vi "Teleop.vi"(10 "Match Info":T1={"Autonomous Elapsed Seconds"=0.0, "TeleOp Elapsed Seconds"=0.0, "Disabled Elapsed Seconds"=0.0, "Visited Autonomous"=FALSE, "Visited TeleOp"=FALSE, "Visited Disabled"=FALSE, "Autonomous Settings"={"Autonomous Style"=enum."Independent", "VI Refnum"=refnum}}, 11 "Call Context":T2) -> ()   [LabVIEW 2016]
doc: "This VI is called for each TeleOp packet received from the DS where the robot is not disabled. It is often used to read from the joysticks and update I/O or to update setpoints for timed control loops. It should complete and return within 20 milliseconds or it may miss DS packets."
uses:
  <vilib>/Rock Robotics/WPI/DriverStation/WPI_DriverStationDerivedRobotMode.ctl
  <vilib>/Rock Robotics/WPI/DriverStation/WPI_DriverStationMatch Info.ctl
  Robot Global Data.vi
  <vilib>/Rock Robotics/WPI/RobotDrive/WPI_RobotDriveArcadeDrive_Standard(NoSaturation).vi
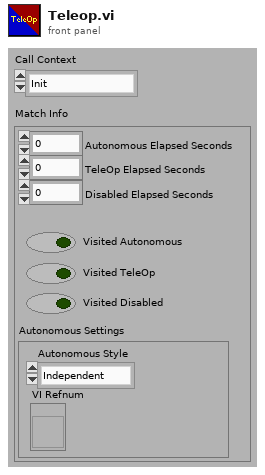
[diagram p1: front panel]
types:
  T1 = typedef "WPI_DriverStationMatch Info.ctl" = cluster{"Autonomous Elapsed Seconds":dbl, "TeleOp Elapsed Seconds":dbl, "Disabled Elapsed Seconds":dbl, "Visited Autonomous":bool, "Visited TeleOp":bool, "Visited Disabled":bool, "Autonomous Settings":cluster{"Autonomous Style":enum16{"Iterative", "Independent"}, "VI Refnum":refnum<vi>}}
  T2 = typedef "WPI_DriverStationDerivedRobotMode.ctl" = enum16{"Init", "Execute", "Stop"}
  T3 = typedef "WPI_RobotDriveDevRef.ctl" = cluster{"DevStatus":errorcluster, "Motors[]":T4[], "Square Inputs":bool, "Max Output":dbl}
  T4 = typedef "WPI_MotorControlDeviceRef.ctl" = cluster{"DeviceStatus":errorcluster, "Type":T5, "PWM":cluster{"PWM Channel":T6, "DeadBand":T7}, "CAN":cluster{"Device Number":u8, "SetOutput VI Ref":variant, "GetOutput VI Ref":variant, "Enable VI Ref":variant, "Disable VI Ref":variant, "Data":variant}, "Invert":bool}
  T5 = typedef "WPI_MotorControlType.ctl" = enum16{"PWM", "CAN"}
  T6 = typedef "FPGA_DIOPWMChannel.ctl" = enum8{"PWM 0", "PWM 1", "PWM 2", "PWM 3", "PWM 4", "PWM 5", "PWM 6", "PWM 7", "PWM 8", "PWM 9", "PWM MXP 0", "PWM MXP 1", "PWM MXP 2", "PWM MXP 3", "PWM MXP 4", "PWM MXP 5", "PWM MXP 6", "PWM MXP 7", "PWM MXP 8", "PWM MXP 9", "Invalid"}
  T7 = typedef "WPI_PWMDeadband.ctl" = cluster{"Name":string, "maxPositivePwm":i32, "minPositivePwm":i32, "centerPwm":i32, "maxNegativePwm":i32, "minNegativePwm":i32, "angularRange":u16}
  T8 = enum16{"Init", "Tank drive", "Right Arcade", "Left Arcade", "Forward", "Vision Alignment", "Stop"}
  T9 = enum16{"Init", "Tank Drive", "Left Arcade", "Right Arcade", "Forward", "Vision Alignment", "Climb", "Stop"}
  T10 = enum16{"Init", "Tank Drive", "Left Arcade", "Right Arcade", "Forward", "Back", "Vision Alignment", "Climb", "Stop"}
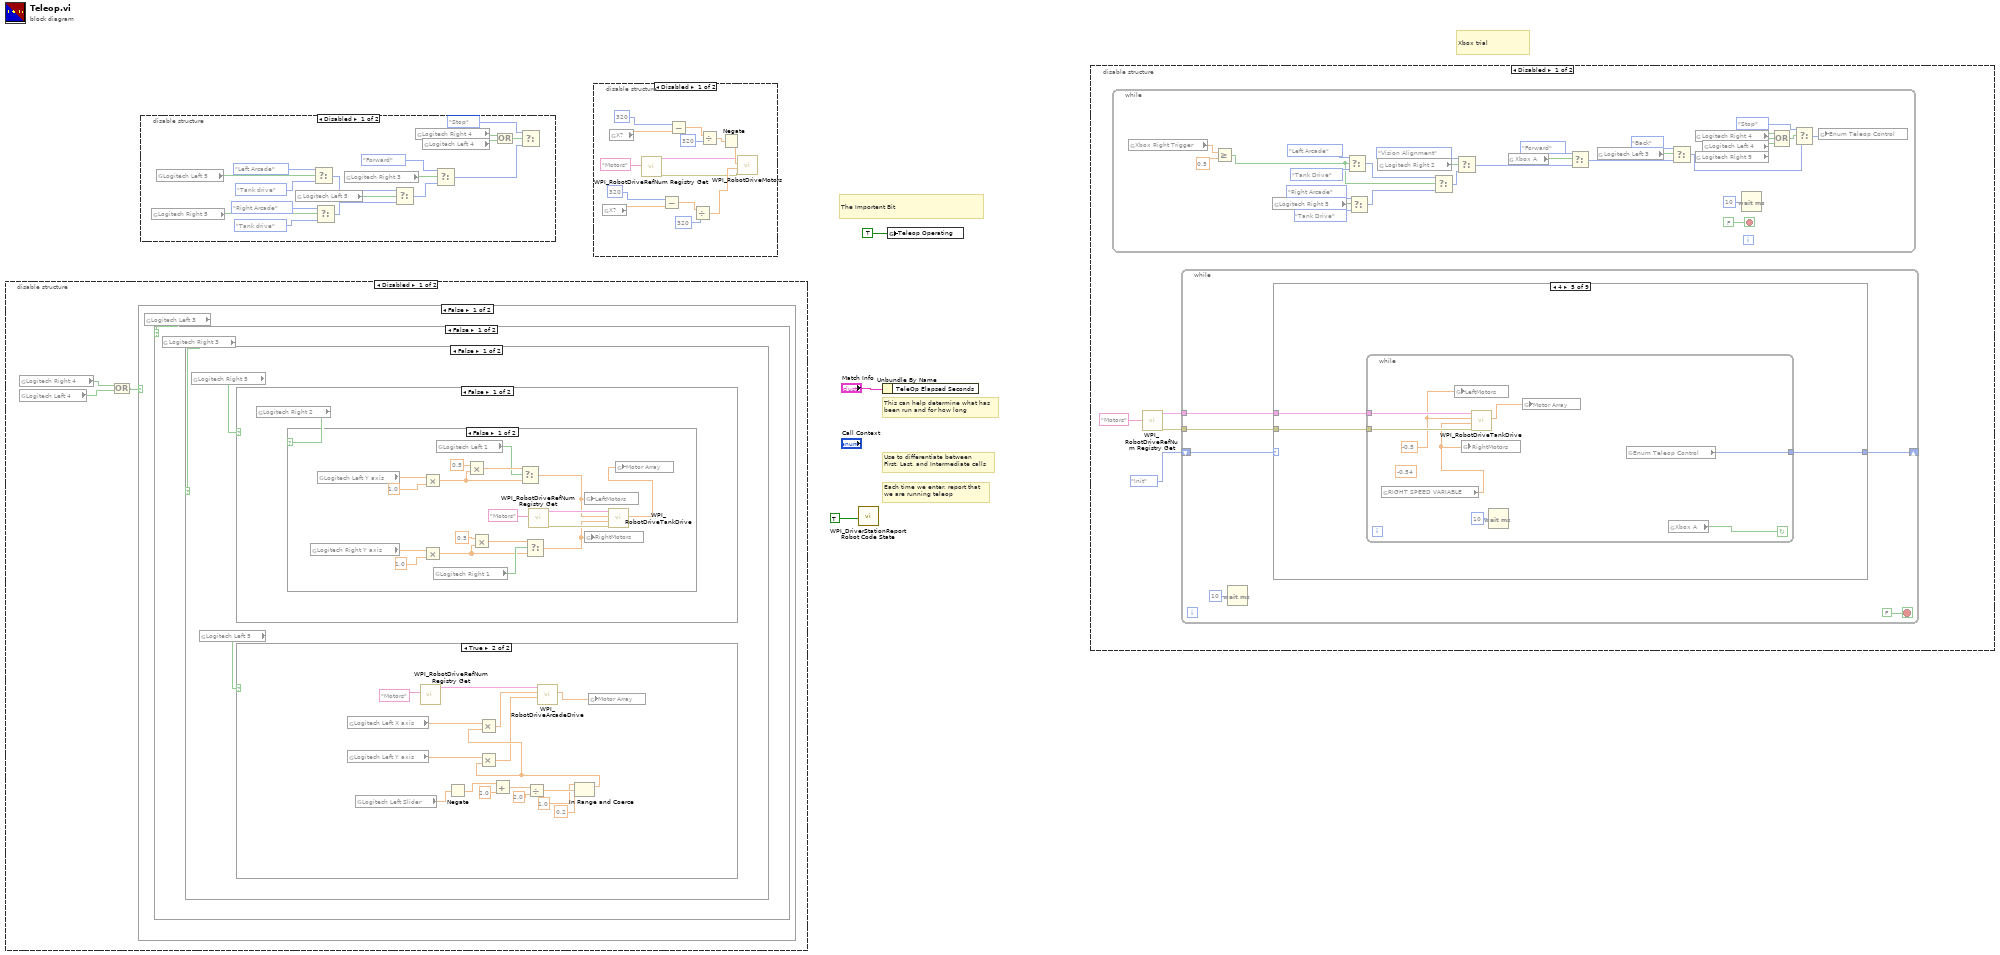
[diagram p0: block diagram]
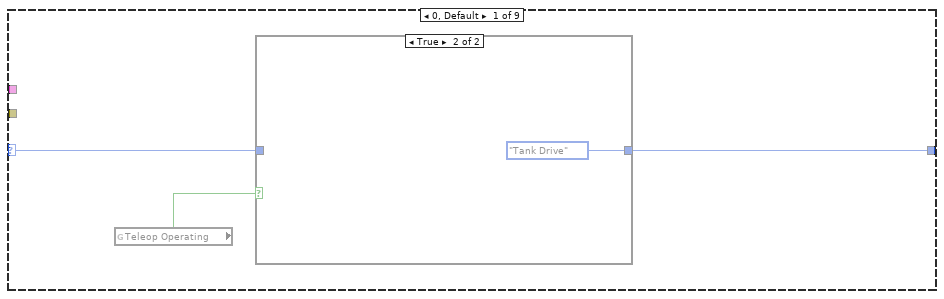
[diagram p2: hidden frame]
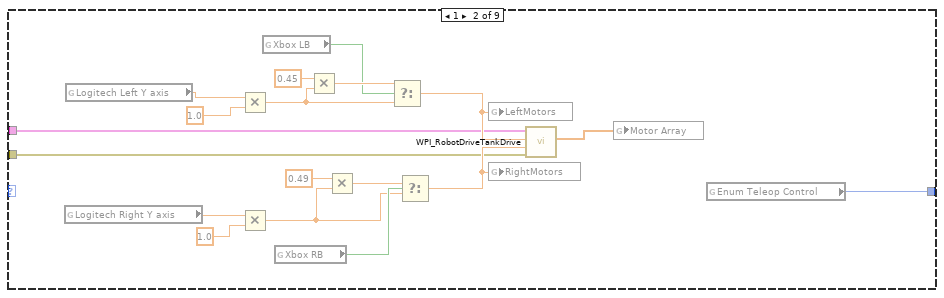
[diagram p4: hidden frame]
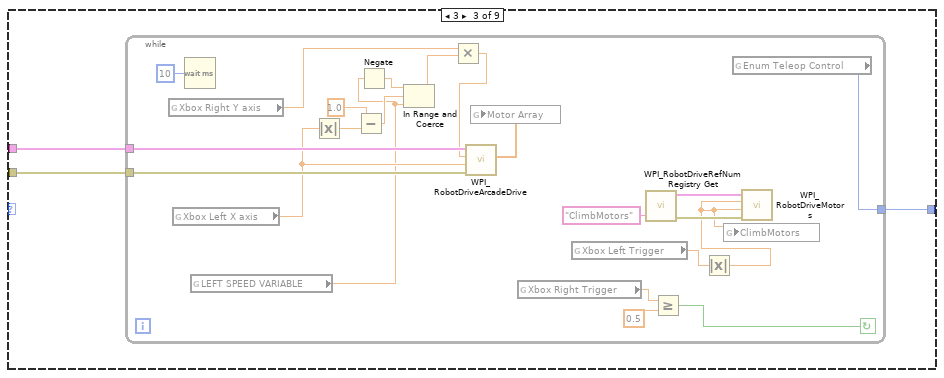
[diagram p5: hidden frame]
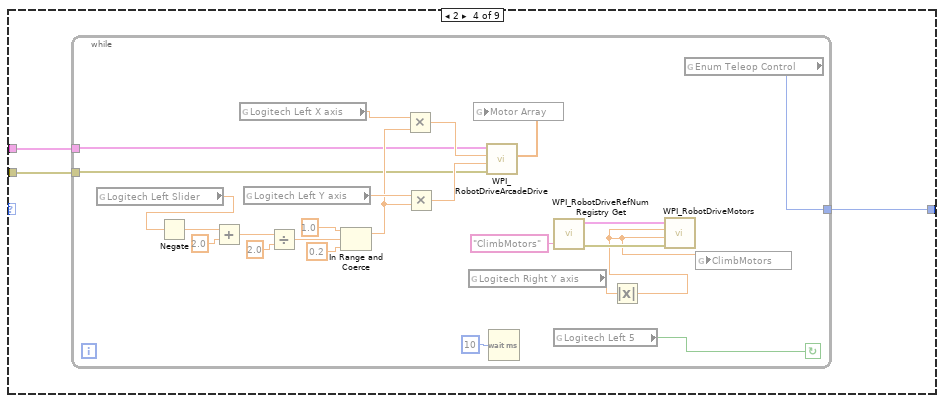
[diagram p6: hidden frame]
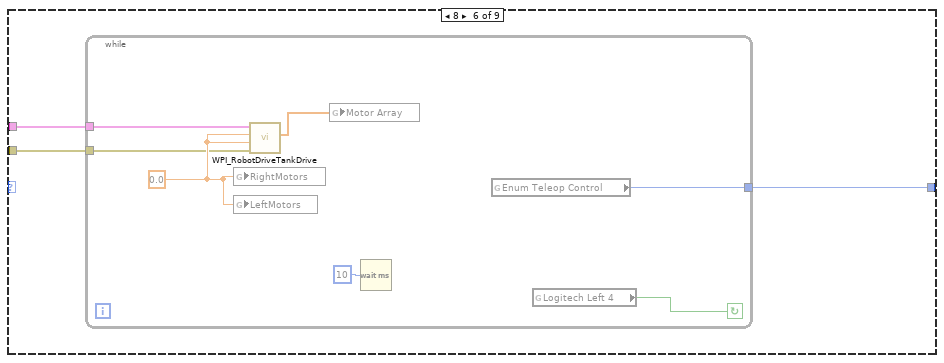
[diagram p7: hidden frame]
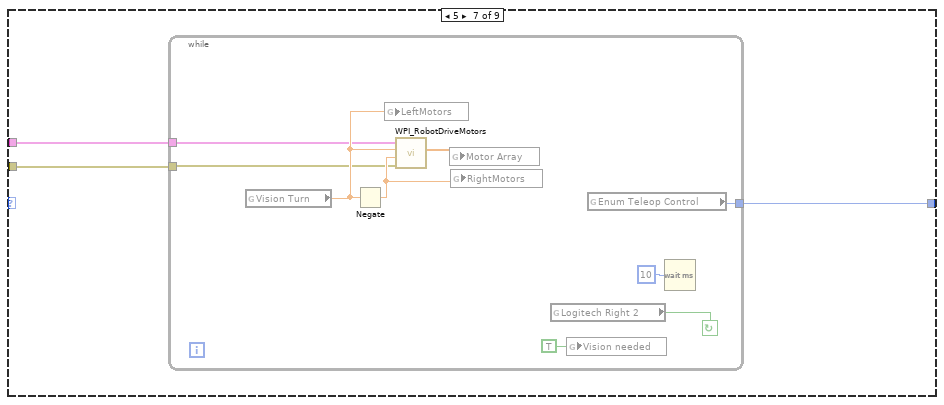
[diagram p8: hidden frame]
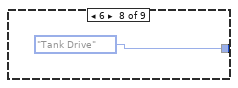
[diagram p9: hidden frame]
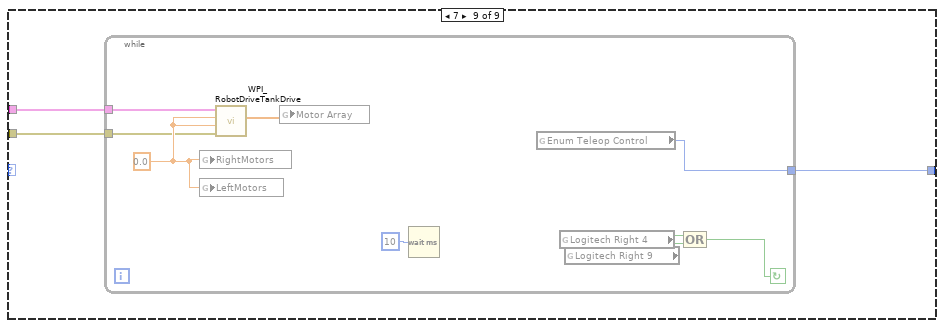
[diagram p10: hidden frame]
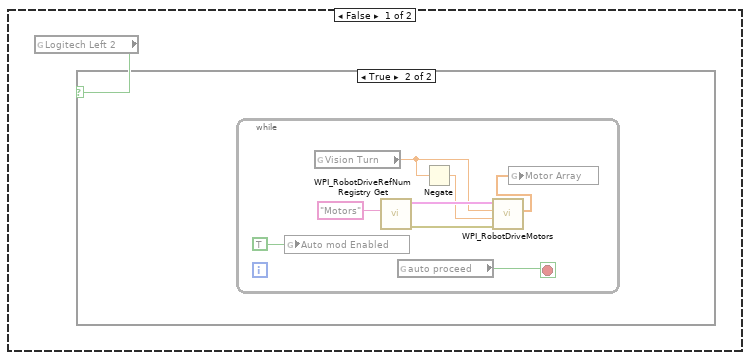
[diagram p12: hidden frame]
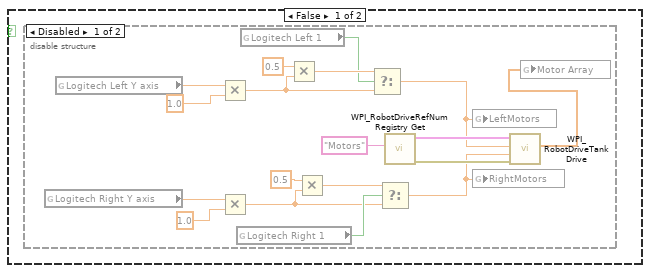
[diagram p13: hidden frame]
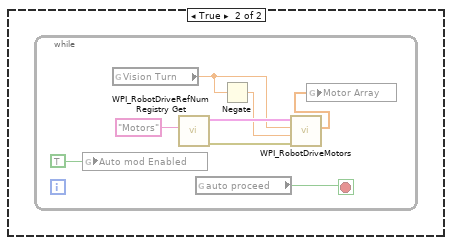
[diagram p15: hidden frame]
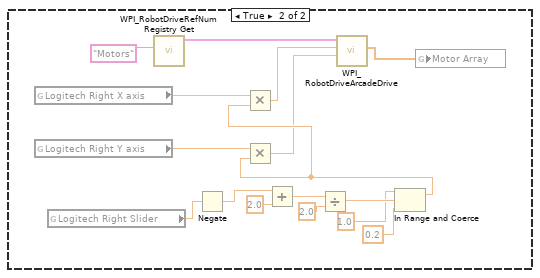
[diagram p16: hidden frame]
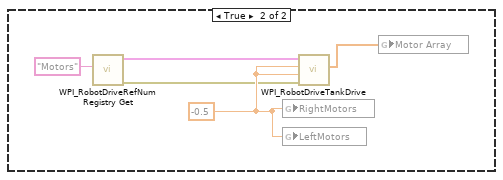
[diagram p17: hidden frame]
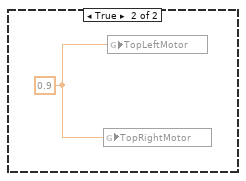
[diagram p18: hidden frame]
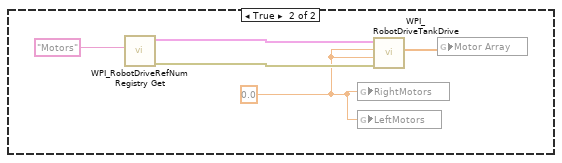
[diagram p19: hidden frame]
diagram:
  # "Xbox trial"
  # "The Importent Bit"
  # "Each time we enter, report that\nwe are running teleop"
  # "Use to differentiate between\nFirst, Last, and Intermediate calls"
  # "This can help determine what has\nbeen run and for how long"
  n1 = disable-structure shown="Disabled" {
    frame Disabled {
      n2 = global read "Robot Global Data.vi" "Logitech Right 4"() -> (w4:bool)
      n3 = global read "Robot Global Data.vi" "Logitech Left 4"() -> (w6:bool)
      n4 = Compound Arithmetic op=OR(w4, w6) -> (w5:bool)
      n5 = case shown="False" w5 {
        frame False {
          n6 = global read "Robot Global Data.vi" "Logitech Left 3"() -> (w7:bool)
          n7 = case shown="False" w7 {
            frame False {
              n8 = global read "Robot Global Data.vi" "Logitech Right 3"() -> (w8:bool)
              n9 = case shown="False" w8 {
                frame False {
                  n10 = global read "Robot Global Data.vi" "Logitech Right 5"() -> (w10:bool)
                  n11 = global read "Robot Global Data.vi" "Logitech Left 5"() -> (w9:bool)
                  n12 = case shown="False" w10 {
                    frame False {
                      n13 = global read "Robot Global Data.vi" "Logitech Right 2"() -> (w54:bool)
                      n14 = case shown="False" w54 {
                        frame False {
                          n15 = global read "Robot Global Data.vi" "Logitech Right Y axis"() -> (w66:dbl)
                          n16 = global read "Robot Global Data.vi" "Logitech Left Y axis"() -> (w69:dbl)
                          n17 = Multiply(x=w69, y=1.0) -> (x*y=w63:dbl)
                          n18 = Multiply(x=w66, y=1.0) -> (x*y=w59:dbl)
                          n19 = global read "Robot Global Data.vi" "Logitech Right 1"() -> (w60:bool)
                          n20 = global read "Robot Global Data.vi" "Logitech Left 1"() -> (w58:bool)
                          n21 = Multiply(x=0.5 ("y"), y=w63) -> (x*y=w64:dbl)
                          n22 = Multiply(x=0.5 ("y"), y=w59) -> (x*y=w62:dbl)
                          n23 = Select(t=w64, s=w58, f=w63) -> (s? t:f=w57:dbl)
                          n24 = Select(t=w62, s=w60, f=w59) -> (s? t:f=w56:dbl)
                          n25 = call <vilib>:"WPI_RobotDriveRefNum Registry Get.vi"("refnum name"="Motors") -> ("error out"=w71:errorcluster, "RobotDriveDevRef"=w72:T3)  [unwired: 9 in]
                          n26 = global write "Robot Global Data.vi" "LeftMotors"(w57) -> ()
                          n27 = global write "Robot Global Data.vi" "RightMotors"(w56) -> ()
                          n28 = call <vilib>:"WPI_RobotDriveTankDrive.vi"("error in (no error)"=w71, "Right axis value"=w56, "Left axis value"=w57, "RobotDriveDevRef"=w72) -> ("Motor Values"=w55:dbl[])  [unwired: 5 in, 2 out]
                          n29 = global write "Robot Global Data.vi" "Motor Array"(w55) -> ()
                        }
                        frame True {
                          n30 = while {
                            stop <- w74 stop-if-true
                            n31 = global write "Robot Global Data.vi" "Auto mod Enabled"(TRUE ("Auto mod Enabled")) -> ()
                            n32 = global read "Robot Global Data.vi" "Vision Turn"() -> (w77:dbl)
                            n33 = call <vilib>:"WPI_RobotDriveRefNum Registry Get.vi"("refnum name"="Motors") -> ("error out"=w78:errorcluster, "RobotDriveDevRef"=w79:T3)  [unwired: 9 in]
                            n34 = global read "Robot Global Data.vi" "auto proceed"() -> (w74:bool)
                            n35 = Negate(x=w77) -> (-x=w76:dbl)
                            n36 = call <vilib>:"WPI_RobotDriveMotors.vi"("error in (no error)"=w78, "RightSpeed"=w76, "LeftSpeed"=w77, "RobotDriveDevRef"=w79) -> ("Motor Values"=w73:dbl[])  [unwired: 7 out]
                            n37 = global write "Robot Global Data.vi" "Motor Array"(w73) -> ()
                          }
                        }
                      }
                    }
                    frame True {
                      n38 = global read "Robot Global Data.vi" "Logitech Right X axis"() -> (w88:dbl)
                      n39 = global read "Robot Global Data.vi" "Logitech Right Y axis"() -> (w87:dbl)
                      n40 = global read "Robot Global Data.vi" "Logitech Right Slider"() -> (w92:dbl)
                      n41 = call <vilib>:"WPI_RobotDriveRefNum Registry Get.vi"("refnum name"="Motors") -> ("RobotDriveDevRef"=w83:T3)  [unwired: 9 in, 1 out]
                      n42 = Negate(x=w92) -> (-x=w91:dbl)
                      n43 = Add(x=w91, y=2.0) -> (x+y=w85:dbl)
                      n44 = Divide(x=w85, y=2.0) -> (x/y=w95:dbl)
                      n45 = In Range and Coerce(upper limit=1.0, x=w95, lower limit=0.2) -> (coerced(x)=w96:dbl)  [unwired: 1 out]
                      n46 = Multiply(x=w88, y=w96) -> (x*y=w89:dbl)
                      n47 = Multiply(x=w87, y=w96) -> (x*y=w90:dbl)
                      n48 = call-poly <vilib>:"WPI_RobotDriveArcadeDrive.vi"("Y axis value"=w90, "X axis value"=w89, "RobotDriveDevRef"=w83) -> ("Motor Values"=w81:dbl[])  [unwired: 6 in, 2 out]
                      n49 = global write "Robot Global Data.vi" "Motor Array"(w81) -> ()
                    }
                  }
                  n50 = case shown="True" w9 {
                    frame False {
                      n51 = global read "Robot Global Data.vi" "Logitech Left 2"() -> (w11:bool)
                      n52 = case shown="True" w11 {
                        frame False {
                          n53 = disable-structure shown="Disabled" {
                            frame Disabled {
                              n54 = global read "Robot Global Data.vi" "Logitech Right Y axis"() -> (w23:dbl)
                              n55 = global read "Robot Global Data.vi" "Logitech Left Y axis"() -> (w26:dbl)
                              n56 = Multiply(x=w26, y=1.0) -> (x*y=w20:dbl)
                              n57 = Multiply(x=w23, y=1.0) -> (x*y=w16:dbl)
                              n58 = global read "Robot Global Data.vi" "Logitech Right 1"() -> (w17:bool)
                              n59 = global read "Robot Global Data.vi" "Logitech Left 1"() -> (w15:bool)
                              n60 = Multiply(x=0.5 ("y"), y=w20) -> (x*y=w21:dbl)
                              n61 = Multiply(x=0.5 ("y"), y=w16) -> (x*y=w19:dbl)
                              n62 = Select(t=w21, s=w15, f=w20) -> (s? t:f=w14:dbl)
                              n63 = Select(t=w19, s=w17, f=w16) -> (s? t:f=w13:dbl)
                              n64 = call <vilib>:"WPI_RobotDriveRefNum Registry Get.vi"("refnum name"="Motors") -> ("error out"=w28:errorcluster, "RobotDriveDevRef"=w29:T3)  [unwired: 9 in]
                              n65 = global write "Robot Global Data.vi" "LeftMotors"(w14) -> ()
                              n66 = global write "Robot Global Data.vi" "RightMotors"(w13) -> ()
                              n67 = call <vilib>:"WPI_RobotDriveTankDrive.vi"("error in (no error)"=w28, "Right axis value"=w13, "Left axis value"=w14, "RobotDriveDevRef"=w29) -> ("Motor Values"=w12:dbl[])  [unwired: 5 in, 2 out]
                              n68 = global write "Robot Global Data.vi" "Motor Array"(w12) -> ()
                            }
                            frame Enabled {
                            }
                          }
                        }
                        frame True {
                          n69 = while {
                            stop <- w31 stop-if-true
                            n70 = global write "Robot Global Data.vi" "Auto mod Enabled"(TRUE ("Auto mod Enabled")) -> ()
                            n71 = global read "Robot Global Data.vi" "Vision Turn"() -> (w34:dbl)
                            n72 = call <vilib>:"WPI_RobotDriveRefNum Registry Get.vi"("refnum name"="Motors") -> ("error out"=w35:errorcluster, "RobotDriveDevRef"=w36:T3)  [unwired: 9 in]
                            n73 = global read "Robot Global Data.vi" "auto proceed"() -> (w31:bool)
                            n74 = Negate(x=w34) -> (-x=w33:dbl)
                            n75 = call <vilib>:"WPI_RobotDriveMotors.vi"("error in (no error)"=w35, "RightSpeed"=w33, "LeftSpeed"=w34, "RobotDriveDevRef"=w36) -> ("Motor Values"=w30:dbl[])  [unwired: 7 out]
                            n76 = global write "Robot Global Data.vi" "Motor Array"(w30) -> ()
                          }
                        }
                      }
                    }
                    frame True {
                      n77 = global read "Robot Global Data.vi" "Logitech Left X axis"() -> (w45:dbl)
                      n78 = global read "Robot Global Data.vi" "Logitech Left Y axis"() -> (w44:dbl)
                      n79 = global read "Robot Global Data.vi" "Logitech Left Slider"() -> (w49:dbl)
                      n80 = call <vilib>:"WPI_RobotDriveRefNum Registry Get.vi"("refnum name"="Motors") -> ("RobotDriveDevRef"=w40:T3)  [unwired: 9 in, 1 out]
                      n81 = Negate(x=w49) -> (-x=w48:dbl)
                      n82 = Add(x=w48, y=2.0) -> (x+y=w42:dbl)
                      n83 = Divide(x=w42, y=2.0) -> (x/y=w52:dbl)
                      n84 = In Range and Coerce(upper limit=1.0, x=w52, lower limit=0.2) -> (coerced(x)=w53:dbl)  [unwired: 1 out]
                      n85 = Multiply(x=w45, y=w53) -> (x*y=w46:dbl)
                      n86 = Multiply(x=w44, y=w53) -> (x*y=w47:dbl)
                      n87 = call-poly <vilib>:"WPI_RobotDriveArcadeDrive.vi"("Y axis value"=w47, "X axis value"=w46, "RobotDriveDevRef"=w40) -> ("Motor Values"=w38:dbl[])  [unwired: 6 in, 2 out]
                      n88 = global write "Robot Global Data.vi" "Motor Array"(w38) -> ()
                    }
                  }
                }
                frame True {
                  w101 = -0.5 ("Right axis value")
                  n89 = call <vilib>:"WPI_RobotDriveRefNum Registry Get.vi"("refnum name"="Motors") -> ("error out"=w99:errorcluster, "RobotDriveDevRef"=w100:T3)  [unwired: 9 in]
                  n90 = global write "Robot Global Data.vi" "RightMotors"(w101) -> ()
                  n91 = global write "Robot Global Data.vi" "LeftMotors"(w101) -> ()
                  n92 = call <vilib>:"WPI_RobotDriveTankDrive.vi"("error in (no error)"=w99, "Right axis value"=w101, "Left axis value"=w101, "RobotDriveDevRef"=w100) -> ("Motor Values"=w97:dbl[])  [unwired: 5 in, 2 out]
                  n93 = global write "Robot Global Data.vi" "Motor Array"(w97) -> ()
                }
              }
            }
            frame True {
              w102 = 0.9
              n94 = global write "Robot Global Data.vi" "TopRightMotor"(w102) -> ()
              n95 = global write "Robot Global Data.vi" "TopLeftMotor"(w102) -> ()
            }
          }
        }
        frame True {
          w104 = 0.0 ("Right axis value")
          n96 = call <vilib>:"WPI_RobotDriveRefNum Registry Get.vi"("refnum name"="Motors") -> ("error out"=w106:errorcluster, "RobotDriveDevRef"=w105:T3)  [unwired: 9 in]
          n97 = global write "Robot Global Data.vi" "RightMotors"(w104) -> ()
          n98 = global write "Robot Global Data.vi" "LeftMotors"(w104) -> ()
          n99 = call <vilib>:"WPI_RobotDriveTankDrive.vi"("error in (no error)"=w106, "Right axis value"=w104, "Left axis value"=w104, "RobotDriveDevRef"=w105) -> ("Motor Values"=w103:dbl[])  [unwired: 5 in, 2 out]
          n100 = global write "Robot Global Data.vi" "Motor Array"(w103) -> ()
        }
      }
    }
    frame Enabled {
    }
  }
  n101 = disable-structure shown="Disabled" {
    frame Disabled {
      n102 = global read "Robot Global Data.vi" "Logitech Right 5"() -> (w117:bool)
      n103 = global read "Robot Global Data.vi" "Logitech Left 5"() -> (w118:bool)
      n104 = global read "Robot Global Data.vi" "Logitech Left 5"() -> (w121:bool)
      n105 = Select(t=T8."Left Arcade", s=w118, f=T8."Tank drive") -> (s? t:f=w120:T8)
      n106 = Select(t=T8."Right Arcade", s=w117, f=T8."Tank drive") -> (s? t:f=w119:T8)
      n107 = global read "Robot Global Data.vi" "Logitech Right 3"() -> (w122:bool)
      n108 = Select(t=w120, s=w121, f=w119) -> (s? t:f=w124:T8)
      n109 = global read "Robot Global Data.vi" "Logitech Right 4"() -> (w110:bool)
      n110 = global read "Robot Global Data.vi" "Logitech Left 4"() -> (w112:bool)
      n111 = Select(t=T8."Forward", s=w122, f=w124) -> (s? t:f=w108:T8)
      n112 = Compound Arithmetic op=OR(w110, w112) -> (w111:bool)
      n113 = Select(t=T8."Stop", s=w111, f=w108) -> ()  [unwired: 1 out]
    }
    frame Enabled {
    }
  }
  n114 = disable-structure shown="Disabled" {
    frame Disabled {
      n115 = global read "Robot Global Data.vi" "X?"() -> (w133:dbl)
      n116 = global read "Robot Global Data.vi" "X?"() -> (w125:dbl)
      n117 = call <vilib>:"WPI_RobotDriveRefNum Registry Get.vi"("refnum name"="Motors") -> ("error out"=w129:errorcluster, "RobotDriveDevRef"=w130:T3)  [unwired: 9 in]
      n118 = Subtract(x=320, y=w133) -> (x-y=w132:dbl)
      n119 = Subtract(x=320, y=w125) -> (x-y=w126:dbl)
      n120 = Divide(x=w132, y=320) -> (x/y=w134:dbl)
      n121 = Divide(x=w126, y=320) -> (x/y=w135:dbl)
      n122 = Negate(x=w135) -> (-x=w136:dbl)
      n123 = call <vilib>:"WPI_RobotDriveMotors.vi"("error in (no error)"=w129, "RightSpeed"=w134, "LeftSpeed"=w136, "RobotDriveDevRef"=w130) -> ()  [unwired: 8 out]
    }
    frame Enabled {
    }
  }
  n124 = call <vilib>:"WPI_DriverStationReport Robot Code State.vi"("TeleOp"=TRUE ("Autonomous")) -> ()  [unwired: 10 in, 1 out]
  n125 = Unbundle By Name("Match Info") -> ()  [unwired: 1 out]
  n126 = global write "Robot Global Data.vi" "Teleop Operating"(TRUE ("Teleop Enabled")) -> ()
  n127 = disable-structure shown="Disabled" {
    frame Disabled {
      n128 = while {
        stop <- FALSE stop-if-true
        n129 = global read "Robot Global Data.vi" "Xbox Right Trigger"() -> (w144:dbl)
        n130 = Greater Or Equal?(x=w144, y=0.5) -> (x >= y?=w143:bool)
        n131 = global read "Robot Global Data.vi" "Logitech Right 5"() -> (w162:bool)
        n132 = Select(t=T9."Left Arcade", s=w143, f=T9."Tank Drive") -> (s? t:f=w153:T9)
        n133 = Select(t=T9."Right Arcade", s=w162, f=T9."Tank Drive") -> (s? t:f=w152:T9)
        n134 = global read "Robot Global Data.vi" "Logitech Right 2"() -> (w163:bool)
        n135 = Select(t=w153, s=w143, f=w152) -> (s? t:f=w160:T9)
        n136 = Select(t=T9."Vision Alignment", s=w163, f=w160) -> (s? t:f=w161:T9)
        n137 = global read "Robot Global Data.vi" "Xbox A"() -> (w164:bool)
        n138 = Select(t=T9."Forward", s=w164, f=w161) -> (s? t:f=w148:T9)
        n139 = global read "Robot Global Data.vi" "Logitech Left 3"() -> (w149:bool)
        n140 = Select(t=T10."Back", s=w149, f=w148) -> (s? t:f=w147:u16)
        n141 = global read "Robot Global Data.vi" "Logitech Right 4"() -> (w165:bool)
        n142 = global read "Robot Global Data.vi" "Logitech Right 9"() -> (w146:bool)
        n143 = global read "Robot Global Data.vi" "Logitech Left 4"() -> (w166:bool)
        n144 = Wait (ms)(milliseconds to wait=u32 10) -> ()  [unwired: 1 out]
        n145 = Compound Arithmetic op=OR(w165, w166, w146) -> (w167:bool)
        n146 = Select(t=T9."Stop", s=w167, f=w147) -> (s? t:f=w168:u16)
        n147 = global write "Robot Global Data.vi" "Enum Teleop Control"(w168) -> ()
      }
      n148 = call <vilib>:"WPI_RobotDriveRefNum Registry Get.vi"("refnum name"="Motors") -> ("error out"=w141:errorcluster, "RobotDriveDevRef"=w142:T3)  [unwired: 9 in]
      n149 = while {
        tunnel: w142 -> [w176]
        tunnel: w141 -> [w175]
        shift-right: [w171] -> _
        shift-left: T9."Init" -> [w172]
        stop <- FALSE stop-if-true
        n150 = Wait (ms)(milliseconds to wait=u32 10) -> ()  [unwired: 1 out]
        n151 = case shown="4" w172 {
          selector: w172 -> [w177 _ _ _ _ _ _ _ _]
          tunnel: w176 -> [_ w184 w202 w227 w253 w265 w275 _ w288]
          tunnel: w175 -> [_ w183 w201 w226 w254 w264 w274 _ w287]
          tunnel: [w178 w182 w200 w225 w252 w263 w273 T9."Tank Drive" w286] -> w171
          frame 0, Default {
            n152 = global read "Robot Global Data.vi" "Teleop Operating"() -> (w179:bool)
            n153 = case shown="True" w179 {
              tunnel: [w180 T9."Tank Drive"] -> w178
              tunnel: w177 -> [w180 _]
              frame False {
              }
              frame True {
              }
            }
          }
          frame 1 {
            n154 = global read "Robot Global Data.vi" "Logitech Right Y axis"() -> (w196:dbl)
            n155 = global read "Robot Global Data.vi" "Logitech Left Y axis"() -> (w199:dbl)
            n156 = Multiply(x=w199, y=1.0) -> (x*y=w193:dbl)
            n157 = Multiply(x=w196, y=1.0) -> (x*y=w189:dbl)
            n158 = global read "Robot Global Data.vi" "Xbox LB"() -> (w188:bool)
            n159 = global read "Robot Global Data.vi" "Xbox RB"() -> (w190:bool)
            n160 = Multiply(x=0.45 ("y"), y=w193) -> (x*y=w194:dbl)
            n161 = Multiply(x=0.49 ("y"), y=w189) -> (x*y=w192:dbl)
            n162 = Select(t=w194, s=w188, f=w193) -> (s? t:f=w187:dbl)
            n163 = Select(t=w192, s=w190, f=w189) -> (s? t:f=w186:dbl)
            n164 = global write "Robot Global Data.vi" "LeftMotors"(w187) -> ()
            n165 = global write "Robot Global Data.vi" "RightMotors"(w186) -> ()
            n166 = call <vilib>:"WPI_RobotDriveTankDrive.vi"("error in (no error)"=w183, "Right axis value"=w186, "Left axis value"=w187, "RobotDriveDevRef"=w184) -> ("Motor Values"=w185:dbl[])  [unwired: 5 in, 2 out]
            n167 = global write "Robot Global Data.vi" "Motor Array"(w185) -> ()
            n168 = global read "Robot Global Data.vi" "Enum Teleop Control"() -> (w182:u16)
          }
          frame 3 {
            n169 = while {
              tunnel: w202 -> [w223]
              tunnel: w201 -> [w222]
              tunnel: [w220] -> w200
              stop <- w203 continue-if-true
              n170 = global read "Robot Global Data.vi" "Xbox Right Y axis"() -> (w215:dbl)
              n171 = global read "Robot Global Data.vi" "Xbox Left X axis"() -> (w219:dbl)
              n172 = Wait (ms)(milliseconds to wait=u32 10) -> ()  [unwired: 1 out]
              n173 = global read "Robot Global Data.vi" "LEFT SPEED VARIABLE"() -> (w211:dbl)
              n174 = Absolute Value(x=w219) -> (abs(x)=w218:dbl)
              n175 = Subtract(x=1.0, y=w218) -> (x-y=w216:dbl)
              n176 = Negate(x=w211) -> (-x=w212:dbl)
              n177 = In Range and Coerce(upper limit=w212, x=w216, lower limit=w211) -> (coerced(x)=w214:dbl)  [unwired: 1 out]
              n178 = Multiply(x=w215, y=w214) -> (x*y=w213:dbl)
              n179 = call-poly <vilib>:"WPI_RobotDriveArcadeDrive.vi"("error in (no error)"=w222, "Y axis value"=w219, "X axis value"=w213, "RobotDriveDevRef"=w223) -> ("Motor Values"=w224:dbl[])  [unwired: 5 in, 2 out]
              n180 = global write "Robot Global Data.vi" "Motor Array"(w224) -> ()
              n181 = global read "Robot Global Data.vi" "Xbox Right Trigger"() -> (w205:dbl)
              n182 = global read "Robot Global Data.vi" "Xbox Left Trigger"() -> (w207:dbl)
              n183 = call <vilib>:"WPI_RobotDriveRefNum Registry Get.vi"("refnum name"="ClimbMotors") -> ("error out"=w208:errorcluster, "RobotDriveDevRef"=w209:T3)  [unwired: 9 in]
              n184 = Greater Or Equal?(x=w205, y=0.5) -> (x >= y?=w203:bool)
              n185 = Absolute Value(x=w207) -> (abs(x)=w206:dbl)
              n186 = global write "Robot Global Data.vi" "ClimbMotors"(w206) -> ()
              n187 = global read "Robot Global Data.vi" "Enum Teleop Control"() -> (w220:u16)
              n188 = call <vilib>:"WPI_RobotDriveMotors.vi"("error in (no error)"=w208, "RightSpeed"=w206, "LeftSpeed"=w206, "RobotDriveDevRef"=w209) -> ()  [unwired: 8 out]
            }
          }
          frame 2 {
            n189 = while {
              tunnel: w227 -> [w238]
              tunnel: w226 -> [w237]
              tunnel: [w233] -> w225
              stop <- w236 continue-if-true
              n190 = global read "Robot Global Data.vi" "Logitech Left Slider"() -> (w234:dbl)
              n191 = Negate(x=w234) -> (-x=w243:dbl)
              n192 = Add(x=w243, y=2.0) -> (x+y=w249:dbl)
              n193 = global read "Robot Global Data.vi" "Logitech Left X axis"() -> (w246:dbl)
              n194 = global read "Robot Global Data.vi" "Logitech Left Y axis"() -> (w247:dbl)
              n195 = Divide(x=w249, y=2.0) -> (x/y=w240:dbl)
              n196 = In Range and Coerce(upper limit=1.0, x=w240, lower limit=0.2) -> (coerced(x)=w239:dbl)  [unwired: 1 out]
              n197 = Multiply(x=w246, y=w239) -> (x*y=w245:dbl)
              n198 = Multiply(x=w247, y=w239) -> (x*y=w244:dbl)
              n199 = global read "Robot Global Data.vi" "Logitech Right Y axis"() -> (w229:dbl)
              n200 = call-poly <vilib>:"WPI_RobotDriveArcadeDrive.vi"("error in (no error)"=w237, "Y axis value"=w244, "X axis value"=w245, "RobotDriveDevRef"=w238) -> ("Motor Values"=w251:dbl[])  [unwired: 5 in, 2 out]
              n201 = global write "Robot Global Data.vi" "Motor Array"(w251) -> ()
              n202 = Wait (ms)(milliseconds to wait=u32 10) -> ()  [unwired: 1 out]
              n203 = call <vilib>:"WPI_RobotDriveRefNum Registry Get.vi"("refnum name"="ClimbMotors") -> ("error out"=w230:errorcluster, "RobotDriveDevRef"=w231:T3)  [unwired: 9 in]
              n204 = global read "Robot Global Data.vi" "Logitech Left 5"() -> (w236:bool)
              n205 = Absolute Value(x=w229) -> (abs(x)=w228:dbl)
              n206 = call <vilib>:"WPI_RobotDriveMotors.vi"("error in (no error)"=w230, "RightSpeed"=w228, "LeftSpeed"=w228, "RobotDriveDevRef"=w231) -> ()  [unwired: 8 out]
              n207 = global read "Robot Global Data.vi" "Enum Teleop Control"() -> (w233:u16)
              n208 = global write "Robot Global Data.vi" "ClimbMotors"(w228) -> ()
            }
          }
          frame 4 {
            n209 = while {
              tunnel: w254 -> [w261]
              tunnel: w253 -> [w260]
              tunnel: [w258] -> w252
              stop <- w259 continue-if-true
              (unwired) -0.54 ("Right axis value")
              w256 = -0.5 ("Right axis value")
              n210 = global read "Robot Global Data.vi" "RIGHT SPEED VARIABLE"() -> (w255:dbl)
              n211 = global write "Robot Global Data.vi" "LeftMotors"(w256) -> ()
              n212 = global write "Robot Global Data.vi" "RightMotors"(w255) -> ()
              n213 = call <vilib>:"WPI_RobotDriveTankDrive.vi"("error in (no error)"=w261, "Right axis value"=w255, "Left axis value"=w256, "RobotDriveDevRef"=w260) -> ("Motor Values"=w262:dbl[])  [unwired: 5 in, 2 out]
              n214 = Wait (ms)(milliseconds to wait=u32 10) -> ()  [unwired: 1 out]
              n215 = global write "Robot Global Data.vi" "Motor Array"(w262) -> ()
              n216 = global read "Robot Global Data.vi" "Enum Teleop Control"() -> (w258:u16)
              n217 = global read "Robot Global Data.vi" "Xbox A"() -> (w259:bool)
            }
          }
          frame 8 {
            n218 = while {
              tunnel: w264 -> [w270]
              tunnel: w265 -> [w269]
              tunnel: [w268] -> w263
              stop <- w266 continue-if-true
              w271 = 0.0 ("Right axis value")
              n219 = global write "Robot Global Data.vi" "RightMotors"(w271) -> ()
              n220 = global write "Robot Global Data.vi" "LeftMotors"(w271) -> ()
              n221 = call <vilib>:"WPI_RobotDriveTankDrive.vi"("error in (no error)"=w270, "Right axis value"=w271, "Left axis value"=w271, "RobotDriveDevRef"=w269) -> ("Motor Values"=w272:dbl[])  [unwired: 5 in, 2 out]
              n222 = global write "Robot Global Data.vi" "Motor Array"(w272) -> ()
              n223 = Wait (ms)(milliseconds to wait=u32 10) -> ()  [unwired: 1 out]
              n224 = global read "Robot Global Data.vi" "Enum Teleop Control"() -> (w268:u16)
              n225 = global read "Robot Global Data.vi" "Logitech Left 4"() -> (w266:bool)
            }
          }
          frame 5 {
            n226 = while {
              tunnel: w275 -> [w277]
              tunnel: w274 -> [w276]
              tunnel: [w284] -> w273
              stop <- w283 continue-if-true
              n227 = global read "Robot Global Data.vi" "Vision Turn"() -> (w279:dbl)
              n228 = Negate(x=w279) -> (-x=w278:dbl)
              n229 = global write "Robot Global Data.vi" "LeftMotors"(w279) -> ()
              n230 = call <vilib>:"WPI_RobotDriveMotors.vi"("error in (no error)"=w276, "RightSpeed"=w278, "LeftSpeed"=w279, "RobotDriveDevRef"=w277) -> ("Motor Values"=w280:dbl[])  [unwired: 7 out]
              n231 = global write "Robot Global Data.vi" "Motor Array"(w280) -> ()
              n232 = global write "Robot Global Data.vi" "RightMotors"(w278) -> ()
              n233 = global read "Robot Global Data.vi" "Logitech Right 2"() -> (w283:bool)
              n234 = global write "Robot Global Data.vi" "Vision needed"(TRUE ("Vision needed")) -> ()
              n235 = global read "Robot Global Data.vi" "Enum Teleop Control"() -> (w284:u16)
              n236 = Wait (ms)(milliseconds to wait=u32 10) -> ()  [unwired: 1 out]
            }
          }
          frame 6 {
          }
          frame 7 {
            n237 = while {
              tunnel: w288 -> [w295]
              tunnel: w287 -> [w294]
              tunnel: [w290] -> w286
              stop <- w291 continue-if-true
              w296 = 0.0 ("Right axis value")
              n238 = global write "Robot Global Data.vi" "RightMotors"(w296) -> ()
              n239 = global write "Robot Global Data.vi" "LeftMotors"(w296) -> ()
              n240 = call <vilib>:"WPI_RobotDriveTankDrive.vi"("error in (no error)"=w294, "Right axis value"=w296, "Left axis value"=w296, "RobotDriveDevRef"=w295) -> ("Motor Values"=w297:dbl[])  [unwired: 5 in, 2 out]
              n241 = global write "Robot Global Data.vi" "Motor Array"(w297) -> ()
              n242 = Wait (ms)(milliseconds to wait=u32 10) -> ()  [unwired: 1 out]
              n243 = global read "Robot Global Data.vi" "Enum Teleop Control"() -> (w290:u16)
              n244 = global read "Robot Global Data.vi" "Logitech Right 4"() -> (w292:bool)
              n245 = global read "Robot Global Data.vi" "Logitech Right 9"() -> (w293:bool)
              n246 = Compound Arithmetic op=OR(w292, w293) -> (w291:bool)
            }
          }
        }
      }
    }
    frame Enabled {
    }
  }
